vi "Load Profile.vi"(0 "Output":bool, 7 "References":T1) -> ()   [LabVIEW 2018]
uses:
  <vilib>/Utility/file.llb/Read Delimited Spreadsheet (DBL).vi
panel:
  out "string":string
  out "subarray 2":dbl[](array[numeric])
  out "subarray":dbl[](array[numeric])
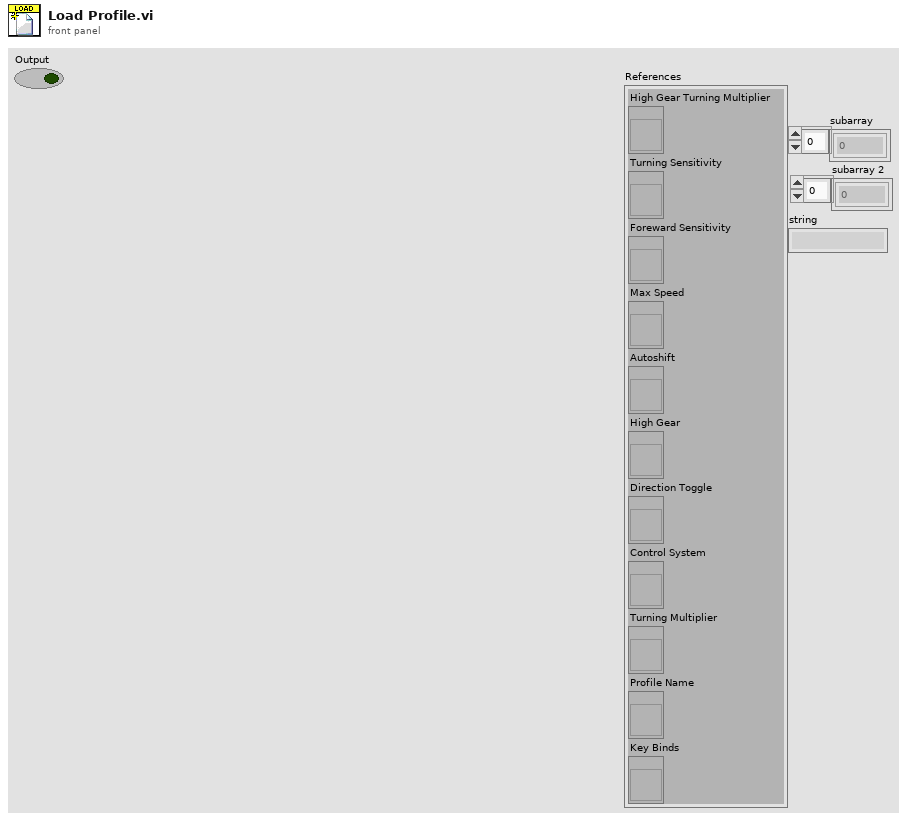
[diagram p1: front panel]
types:
  T1 = cluster{"High Gear Turning Multiplier":refnum<vi>, "Turning Sensitivity":refnum<vi>, "Foreward Sensitivity":refnum<vi>, "Max Speed":refnum<vi>, "Autoshift":refnum<vi>, "High Gear":refnum<vi>, "Direction Toggle":refnum<vi>, "Control System":refnum<vi>, "Turning Multiplier":refnum<vi>, "Profile Name":refnum<vi>, "Key Binds":refnum<vi>}
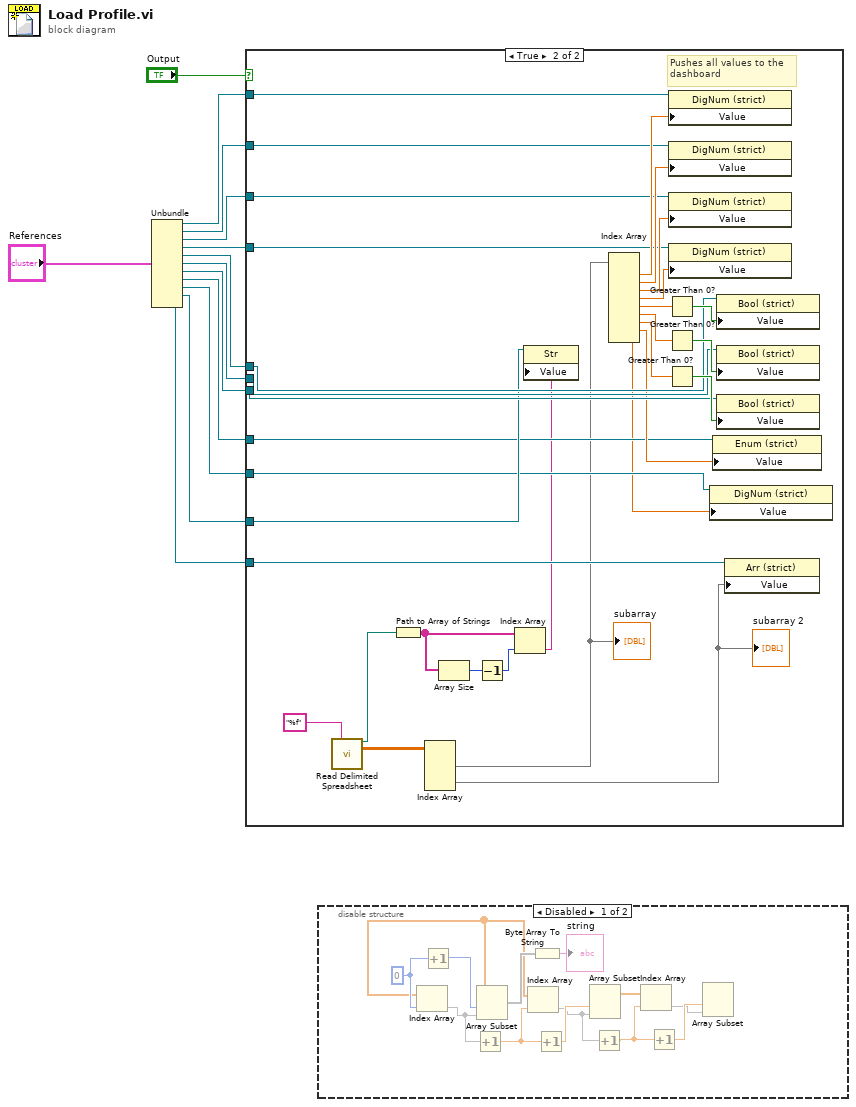
[diagram p0: block diagram]
diagram:
  n1 = Unbundle("References") -> ("High Gear Turning Multiplier"=w12:refnum<vi>, "Turning Sensitivity"=w11:refnum<vi>, "Foreward Sensitivity"=w10:refnum<vi>, "Max Speed"=w9:refnum<vi>, "Autoshift"=w8:refnum<vi>, "High Gear"=w7:refnum<vi>, "Direction Toggle"=w6:refnum<vi>, "Control System"=w5:refnum<vi>, "Turning Multiplier"=w3:refnum<vi>, "Profile Name"=w4:refnum<vi>, "Key Binds"=w1:refnum<vi>)
  n2 = case shown="True" "Output" {
    tunnel: w8 -> [_ w35]
    tunnel: w7 -> [_ w34]
    tunnel: w6 -> [_ w33]
    tunnel: w9 -> [_ w32]
    tunnel: w10 -> [_ w31]
    tunnel: w11 -> [_ w30]
    tunnel: w12 -> [_ w29]
    tunnel: w4 -> [_ w28]
    tunnel: w5 -> [_ w26]
    tunnel: w3 -> [_ w25]
    tunnel: w1 -> [_ w22]
    frame False {
    }
    frame True {
      # "Pushes all values to the \ndashboard"
      n3 = call-poly <vilib>:"Read Delimited Spreadsheet.vi"("format (%.3f)"="%f") -> ("new file path (Not A Path if cancelled)"=w15:path, "all rows"=w21:dbl[][])  [unwired: 9 in, 4 out]
      n4 = Path to Array of Strings(0:w15) -> (2:w18:string[])  [unwired: 1 out]
      n5 = Index Array(array=w21) -> (element #1=w20:dbl[], element #2=w19:dbl[])  [unwired: 4 in]
      "subarray" <- w20
      "subarray 2" <- w19
      n6 = Array Size(array=w18) -> (size(s)=w17:i32)
      n7 = Decrement(x=w17) -> (x-1=w16:i32)
      n8 = Index Array(array=w18, index=w16) -> (element=w14:string)
      n9 = property on="Property Node" class="Str"(reference=w28, "Value"=w14) -> ()  [unwired: 1 in, 2 out]
      n10 = Index Array(array=w20) -> (element #1=w45:dbl, element #2=w44:dbl, element #3=w43:dbl, element #4=w42:dbl, element #5=w41:dbl, element #6=w40:dbl, element #7=w39:dbl, element #8=w27:dbl, element #9=w24:dbl)  [unwired: 9 in]
      n11 = Greater Than 0?(x=w41) -> (x > 0?=w36:bool)
      n12 = Greater Than 0?(x=w40) -> (x > 0?=w37:bool)
      n13 = Greater Than 0?(x=w39) -> (x > 0?=w38:bool)
      n14 = property on="Property Node" class="DigNum (strict)"(reference=w29, "Value"=w45) -> ()  [unwired: 1 in, 2 out]
      n15 = property on="Property Node" class="DigNum (strict)"(reference=w30, "Value"=w44) -> ()  [unwired: 1 in, 2 out]
      n16 = property on="Property Node" class="DigNum (strict)"(reference=w31, "Value"=w43) -> ()  [unwired: 1 in, 2 out]
      n17 = property on="Property Node" class="DigNum (strict)"(reference=w32, "Value"=w42) -> ()  [unwired: 1 in, 2 out]
      n18 = property on="Property Node" class="DigNum (strict)"(reference=w25, "Value"=w24) -> ()  [unwired: 1 in, 2 out]
      n19 = property on="Property Node" class="Enum (strict)"(reference=w26, "Value"=w27) -> ()  [unwired: 1 in, 2 out]
      n20 = property on="Property Node" class="Bool (strict)"(reference=w35, "Value"=w36) -> ()  [unwired: 1 in, 2 out]
      n21 = property on="Property Node" class="Bool (strict)"(reference=w34, "Value"=w37) -> ()  [unwired: 1 in, 2 out]
      n22 = property on="Property Node" class="Bool (strict)"(reference=w33, "Value"=w38) -> ()  [unwired: 1 in, 2 out]
      n23 = property on="Property Node" class="Arr (strict)"(reference=w22, "Value"=w19) -> ()  [unwired: 1 in, 2 out]
    }
  }
  n24 = disable-structure shown="Disabled" {
    frame Disabled {
      w52 = 0 ("index")
      n25 = Increment(x=w52) -> (x+1=w61:i32)
      n26 = Index Array(array=w51, index=w52) -> (element=w59)
      n27 = Increment(x=w59) -> (x+1=w58:dbl)
      n28 = Array Subset(index=w61, length=w59) -> (array=w51:dbl[], w60:void[])
      n29 = Index Array(array=w51, index=w58) -> (element=w53)
      n30 = Byte Array To String(unsigned byte array=w60) -> (string=→"string":string)
      n31 = Increment(x=w58) -> (x+1=w55:dbl)
      n32 = Array Subset(index=w55, length=w53) -> (array=w46:dbl[], w48:void[])
      n33 = Increment(x=w53) -> (x+1=w54:dbl)
      n34 = Index Array(array=w46, index=w54) -> (element=w56)
      n35 = Increment(x=w54) -> (x+1=w57:dbl)
      n36 = Array Subset(index=w57, length=w56) -> (array=w47:dbl[], w49:void[])
    }
    frame Enabled {
    }
  }
